vi "To XML (Core).vi"(8 "error in (no error)":errorcluster, 10 "Parent":refnum<k20>, 11 "Test Suite in":refnum<class "Test Suite.lvclass">) -> (0 "error out":errorcluster)   [LabVIEW 2013, in "JUnit XML.lvlib" / "Test Suite.lvclass"]
doc: "Serializes a Test Suite using NI XML Parser."
uses:
  Test Suite.lvclass
  JUnit XML.lvlib
  <vilib>/xml/NI_XML.lvlib
  <vilib>/xml/Close Reference(Node).vi
  Test Case/Test Result.ctl
  Test Case/Test Case.lvclass
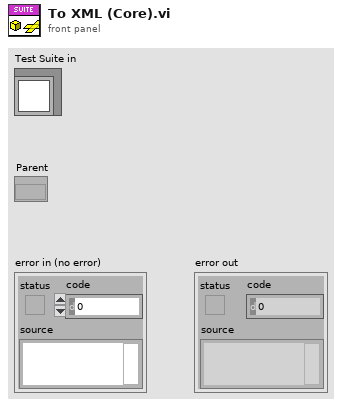
[diagram p1: front panel]
types:
  T1 = typedef "JUnit XML.lvlib/Test Case.lvclass/Test Result.ctl" = enum16{"Success", "Failure", "Error", "Skipped"}
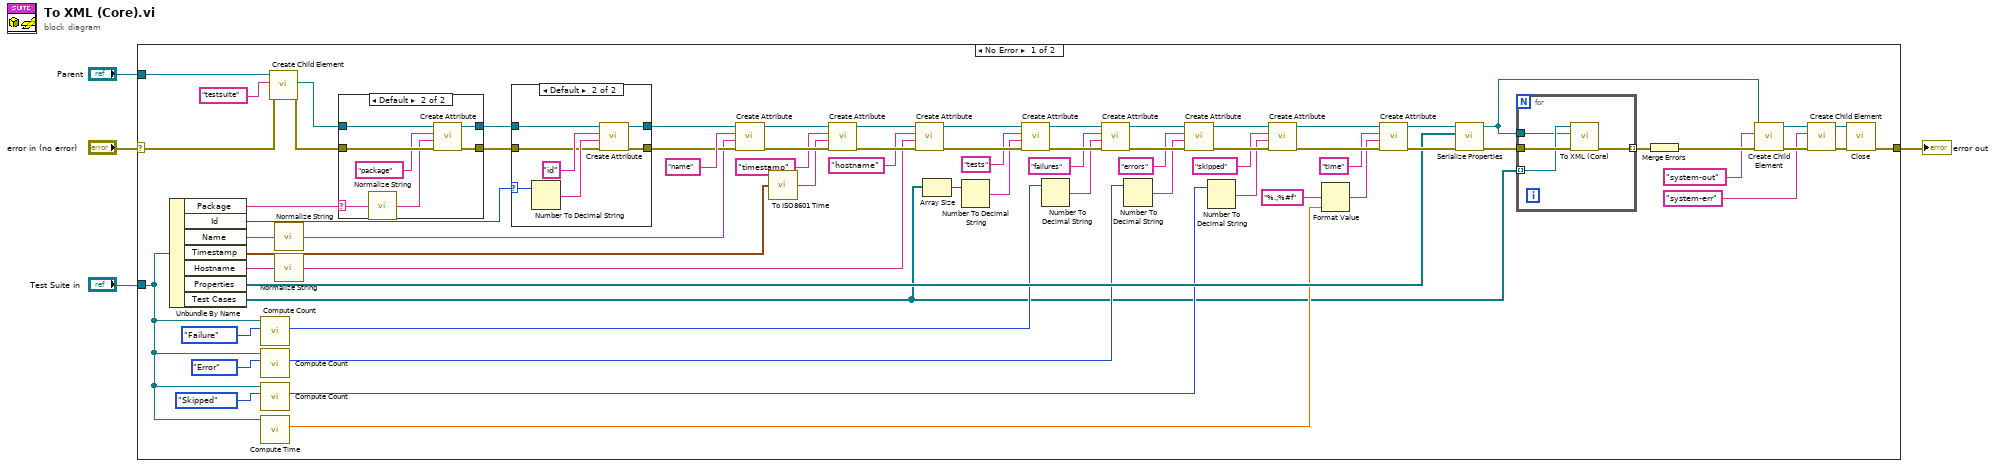
[diagram p0: block diagram]
diagram:
  n1 = case shown="No Error" "error in (no error)" {
    selector: "error in (no error)" -> [w34 w96]
    tunnel: [w22 w96] -> w3
    tunnel: "Test Suite in" -> [w14 _]
    tunnel: "Parent" -> [w33 _]
    frame No Error {
      n2 = Unbundle By Name(w14) -> ("Package"=w5:string, "Id"=w6:i32, "Name"=w71:string, "Timestamp"=w67:timestamp, "Hostname"=w39:string, "Properties"=w21:refnum<class "Property.lvclass">[], "Test Cases"=w10:refnum<class "Test Case.lvclass">[])
      n3 = call "Compute Count.vi"("Test Result"=Test_Result."Failure", "Test Suite in"=w14) -> ("Count"=w12:i32)  [unwired: 7 in, 2 out]
      n4 = call "Compute Count.vi"("Test Result"=Test_Result."Error", "Test Suite in"=w14) -> ("Count"=w13:i32)  [unwired: 7 in, 2 out]
      n5 = call "Compute Count.vi"("Test Result"=Test_Result."Skipped", "Test Suite in"=w14) -> ("Count"=w18:i32)  [unwired: 7 in, 2 out]
      n6 = call "Compute Time.vi"("Test Suite in"=w14) -> ("Time"=w19:dbl)  [unwired: 8 in, 2 out]
      n7 = call "Create Child Element.vi"("error in (no error)"=w34, "Name"="testsuite" ("Tag Name"), "Node in"=w33) -> ("error out"=w37:errorcluster, "Child Element"=w36:refnum<k20>)  [unwired: 6 in, 1 out]
      n8 = call "Normalize String.vi"("String"=w71) -> ("Normalized String"=w9:string)  [unwired: 1 in]
      n9 = call "Normalize String.vi"("String"=w39) -> ("Normalized String"=w8:string)  [unwired: 1 in]
      n10 = case shown="Default" w5 {
        selector: w5 -> [_ w76]
        tunnel: [w74 w82] -> w38
        tunnel: w37 -> [w74 w81]
        tunnel: w36 -> [w75 w80]
        tunnel: [w75 w79] -> w35
        frame "" {
        }
        frame Default {
          n11 = call "Normalize String.vi"("String"=w76) -> ("Normalized String"=w77:string)  [unwired: 1 in]
          n12 = call "Create Attribute.vi"("error in (no error)"=w81, "Value"=w77, "Name"="package" ("Attribute Name"), "Element in"=w80) -> ("error out"=w82:errorcluster, "Element out"=w79:refnum<k20>)  [unwired: 6 in]
        }
      }
      n13 = case shown="Default" w6 {
        selector: w6 -> [_ w85]
        tunnel: [w83 w91] -> w41
        tunnel: [w84 w90] -> w40
        tunnel: w38 -> [w83 w87]
        tunnel: w35 -> [w84 w86]
        frame ..-1 {
        }
        frame Default {
          n14 = Number To Decimal String(number=w85) -> (decimal integer string=w88:string)  [unwired: 1 in]
          n15 = call "Create Attribute.vi"("error in (no error)"=w87, "Value"=w88, "Name"="id" ("Attribute Name"), "Element in"=w86) -> ("error out"=w91:errorcluster, "Element out"=w90:refnum<k20>)  [unwired: 6 in]
        }
      }
      n16 = call "Create Attribute.vi"("error in (no error)"=w41, "Value"=w9, "Name"="name" ("Attribute Name"), "Element in"=w40) -> ("error out"=w69:errorcluster, "Element out"=w70:refnum<k20>)  [unwired: 6 in]
      n17 = call "To ISO8601 Time.vi"("Time Stamp"=w67) -> ("String"=w66:string)  [unwired: 1 in]
      n18 = call "Create Attribute.vi"("error in (no error)"=w69, "Value"=w66, "Name"="timestamp" ("Attribute Name"), "Element in"=w70) -> ("error out"=w64:errorcluster, "Element out"=w65:refnum<k20>)  [unwired: 6 in]
      n19 = call "Create Attribute.vi"("error in (no error)"=w64, "Value"=w8, "Name"="hostname" ("Attribute Name"), "Element in"=w65) -> ("error out"=w61:errorcluster, "Element out"=w62:refnum<k20>)  [unwired: 6 in]
      n20 = Array Size(array=w10) -> (size(s)=w11:i32)
      n21 = Number To Decimal String(number=w11) -> (decimal integer string=w59:string)  [unwired: 1 in]
      n22 = call "Create Attribute.vi"("error in (no error)"=w61, "Value"=w59, "Name"="tests" ("Attribute Name"), "Element in"=w62) -> ("error out"=w58:errorcluster, "Element out"=w57:refnum<k20>)  [unwired: 6 in]
      n23 = Number To Decimal String(number=w12) -> (decimal integer string=w55:string)  [unwired: 1 in]
      n24 = call "Create Attribute.vi"("error in (no error)"=w58, "Value"=w55, "Name"="failures" ("Attribute Name"), "Element in"=w57) -> ("error out"=w53:errorcluster, "Element out"=w54:refnum<k20>)  [unwired: 6 in]
      n25 = Number To Decimal String(number=w13) -> (decimal integer string=w51:string)  [unwired: 1 in]
      n26 = call "Create Attribute.vi"("error in (no error)"=w53, "Value"=w51, "Name"="errors" ("Attribute Name"), "Element in"=w54) -> ("error out"=w49:errorcluster, "Element out"=w50:refnum<k20>)  [unwired: 6 in]
      n27 = Number To Decimal String(number=w18) -> (decimal integer string=w47:string)  [unwired: 1 in]
      n28 = call "Create Attribute.vi"("error in (no error)"=w49, "Value"=w47, "Name"="skipped" ("Attribute Name"), "Element in"=w50) -> ("error out"=w45:errorcluster, "Element out"=w46:refnum<k20>)  [unwired: 6 in]
      n29 = Format Value(format string="%.;%#f", value (0)=w19) -> (output string=w42:string)  [unwired: 1 in]
      n30 = call "Create Attribute.vi"("error in (no error)"=w45, "Value"=w42, "Name"="time" ("Attribute Name"), "Element in"=w46) -> ("error out"=w23:errorcluster, "Element out"=w20:refnum<k20>)  [unwired: 6 in]
      n31 = call "Serialize Properties.vi"("error in (no error)"=w23, "Properties"=w21, "Node in"=w20) -> ("error out"=w31:errorcluster, "Node out"=w7:refnum<k20>)  [unwired: 7 in]
      n32 = for {
        tunnel: [w95] -> w32 mode=indexing
        tunnel: w31 -> [w94]
        tunnel: w10 -> [w93] mode=indexing
        tunnel: w7 -> [w92]
        n33 = call-dynamic "To XML (Core).vi"("error in (no error)"=w94, "Parent"=w92, "Test Case in"=w93) -> ("error out"=w95:errorcluster)  [unwired: 8 in]
      }
      n34 = Merge Errors(w32) -> (w30:errorcluster)
      n35 = call "Create Child Element.vi"("error in (no error)"=w30, "Name"="system-out" ("Tag Name"), "Node in"=w7) -> ("error out"=w28:errorcluster, "Node out"=w29:refnum<k20>)  [unwired: 6 in, 1 out]
      n36 = call "Create Child Element.vi"("error in (no error)"=w28, "Name"="system-err" ("Tag Name"), "Node in"=w29) -> ("error out"=w27:errorcluster, "Node out"=w26:refnum<k20>)  [unwired: 6 in, 1 out]
      n37 = call-poly <vilib>:"Close.vi"("error in (no error)"=w27, "node"=w26) -> ("error out"=w22:errorcluster)  [unwired: 7 in]
    }
    frame Error {
    }
  }
  "error out" <- w3
